vi "Arduino_Timed_Release.vi"(2 "Time to hold source ON (microseconds)":u32=1000000 format="%.0g", 3 "Time to hold source OFF (microseconds)":u32=1000000 format="%.0g", 4 "Number of cycles":u16=1) -> (0 "error out":errorcluster, 1 "Completed cycles":u16=5)   [LabVIEW 2022 SP3]
uses:
  ADAM Serial/Instrument drivers/Arduino/ctls_and_globals/Arduino Config & resource typedef.ctl
  ADAM Client/Sub VIs/ADAM Controls/Update_scan_value.ctl
  <vilib>/Utility/error.llb/Trim Whitespace One-Sided.vi
  Globals/Preference_global.vi
  Globals/Gas_management_global.vi
  Arduino_common/Arduino_comms_Global.vi
panel:
  out "element":T1={"baud rate (bps)"=276000, "timeout (ms)"=12000, "data bits"=8, "parity"=enum."None", "stop bits (10: 1 bit)"=10, "flow control"=0, "termination char (hex)"=10, "Enable Termination Char"=FALSE, "byte count"=12, "Resource locked?"=FALSE, "VISA resource name"=""} {"termination char (hex)" format="%02x"; "stop bits (10: 1 bit)" items=["1.0"=10, "1.5"=15, "2.0"=20]; "flow control" items=["None", "XON/XOFF", "RTS/CTS", "XON/XOFF & RTS/CTS", "DTR/DSR", "XON/XOFF & DTR/DSR"]}
  in  "Device index":i32
  out "bytes sent":u32=12
  out "write buffer":string
  # "(enter 0 for continuous ON)*"
  # "(enter 0 for continuous OFF)*"
  # "Paul Nathan, 18/06/2013, 02/05/2014, 12/08/2014, 03/10/2014, 10/12/2014"
  # "*until next communication. Ensure n cycles is 1 for these special operations."
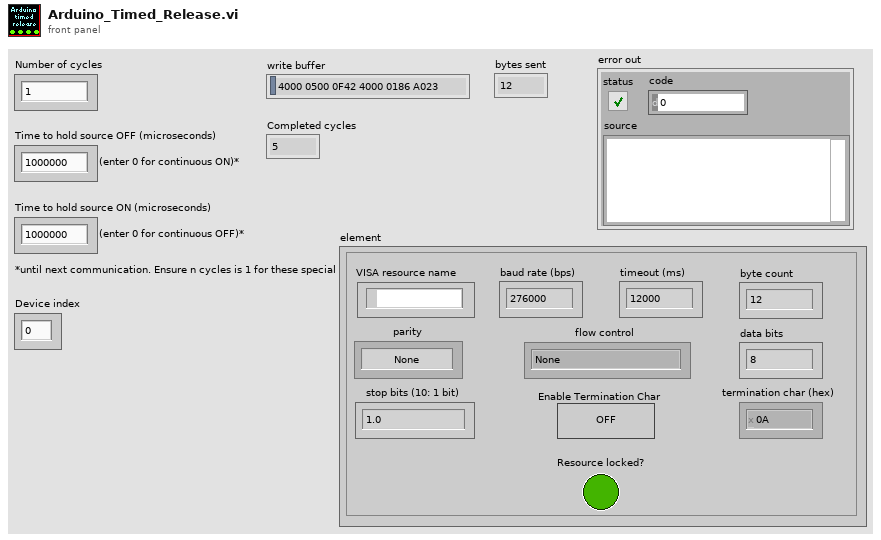
[diagram p1: front panel]
types:
  T1 = typedef "Arduino Config & resource typedef.ctl" = cluster{"baud rate (bps)":u32, "timeout (ms)":u32, "data bits":u16, "parity":enum16{"None", "Odd", "Even", "Mark", "Space"}, "stop bits (10: 1 bit)":u16, "flow control":u16, "termination char (hex)":u8, "Enable Termination Char":bool, "byte count":u32, "Resource locked?":bool, "VISA resource name":refnum<visa-resource-name>}
  T2 = cluster{"Rig Setup":string, "Device index":i32, "Number of cycles":u16, "Time to hold source OFF (microseconds)":u32, "Time to hold source ON (microseconds)":u32}
  T3 = typedef "Update_scan_value.ctl" = cluster{"Channel Name":string, "New Value":dbl, "!Auto_Off":bool}
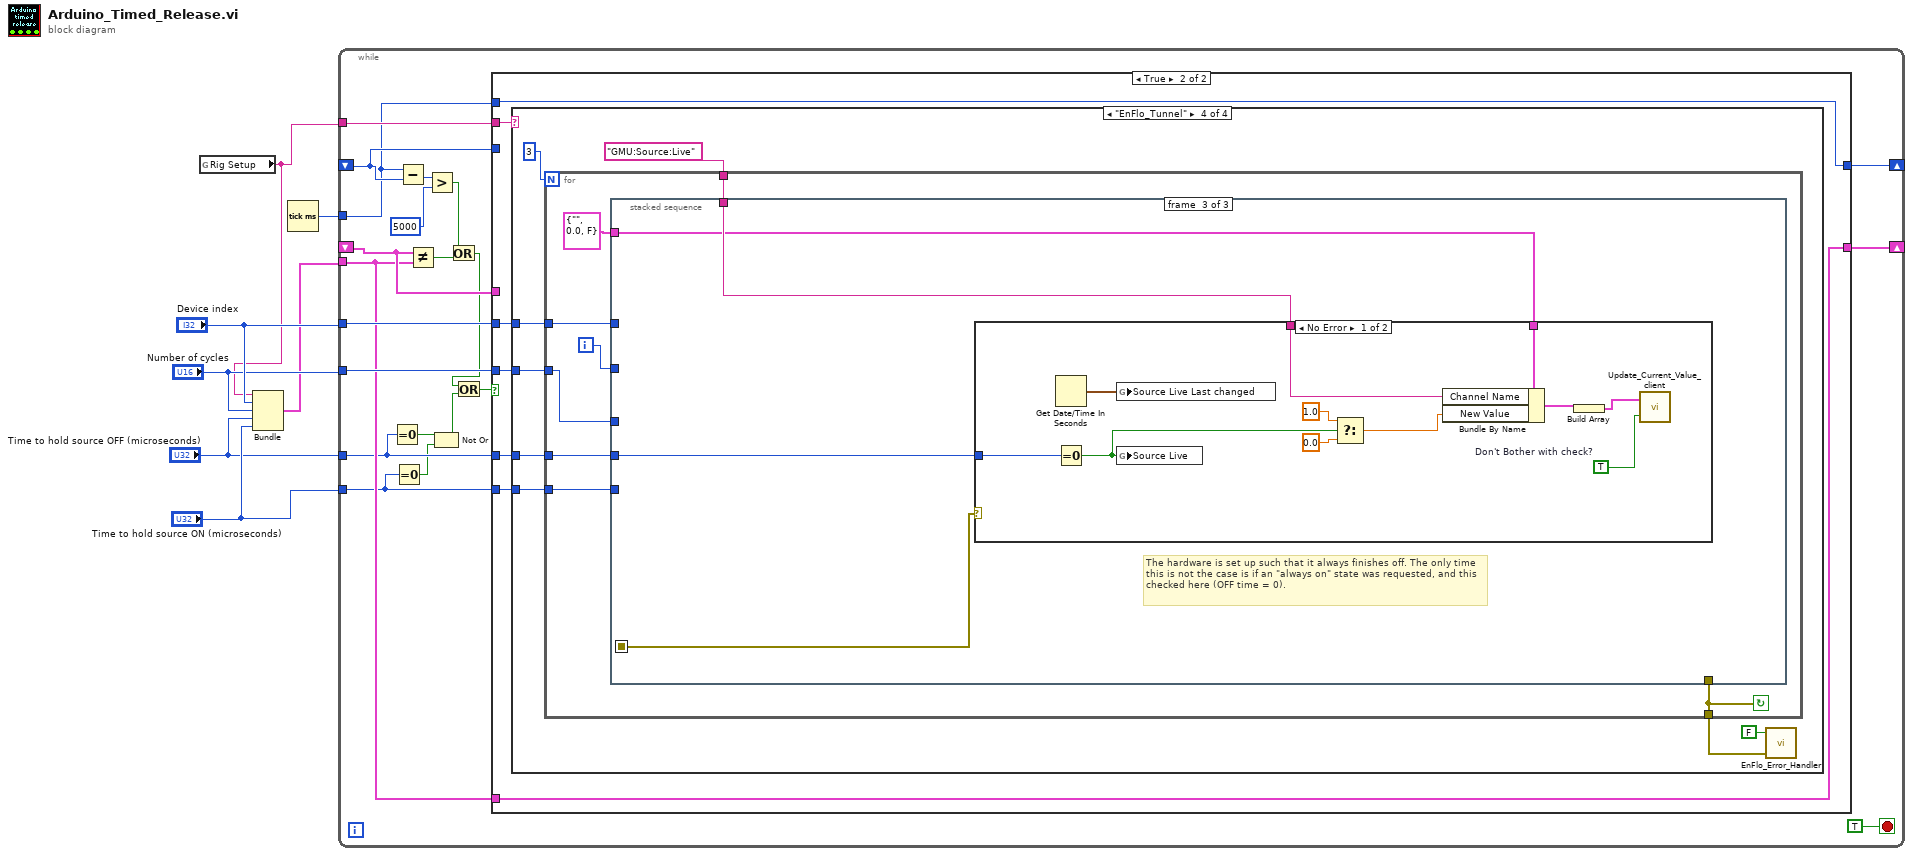
[diagram p0: block diagram]
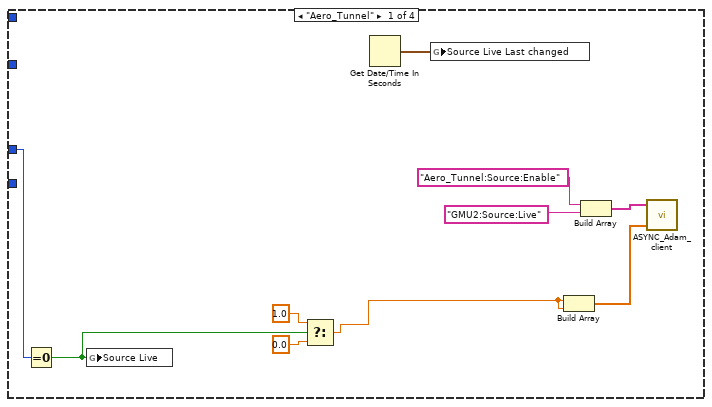
[diagram p3: hidden frame]
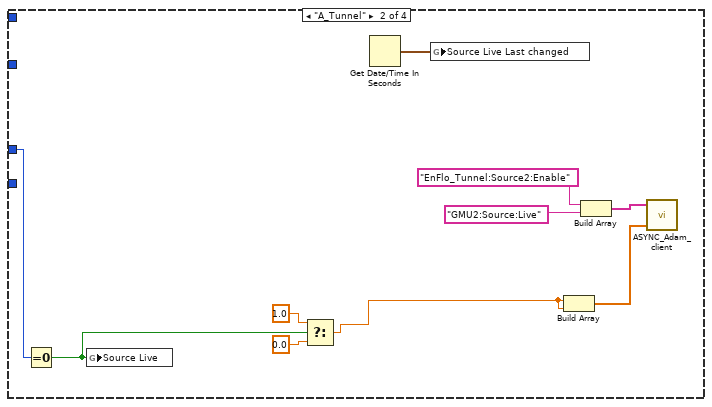
[diagram p4: hidden frame]
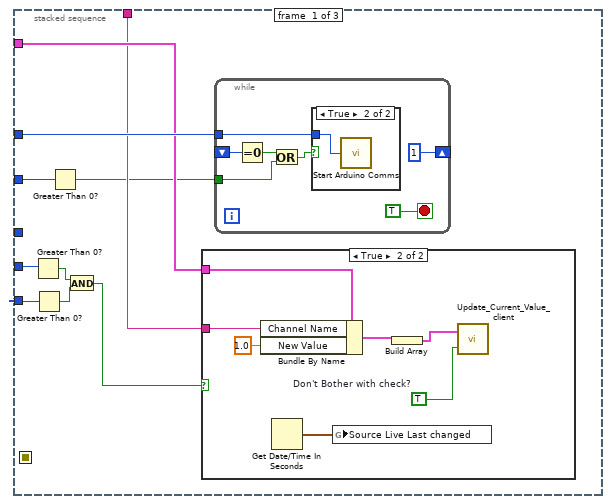
[diagram p6: hidden frame]
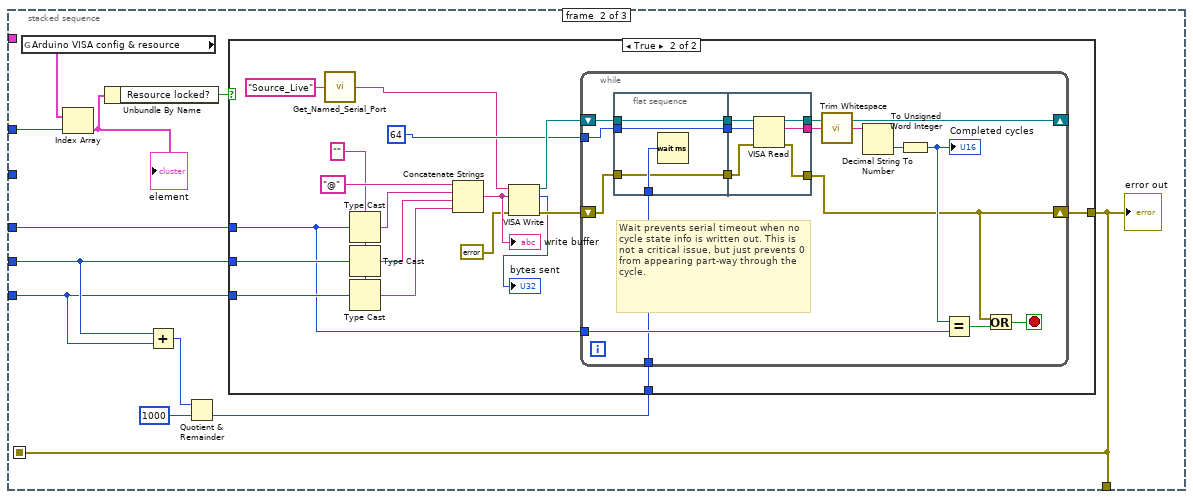
[diagram p9: hidden frame]
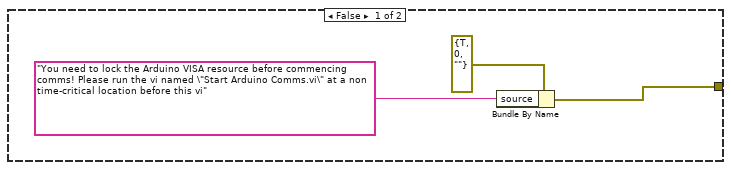
[diagram p10: hidden frame]
diagram:
  n1 = global read "Preference_global.vi" "Rig Setup"() -> (w4:string)
  n2 = Bundle("Rig Setup"=w4, "Device index"="Device index", "Number of cycles"="Number of cycles", "Time to hold source OFF (microseconds)"="Time to hold source OFF (microseconds)", "Time to hold source ON (microseconds)"="Time to hold source ON (microseconds)") -> (w5:T2)  [unwired: 1 in]
  n3 = Tick Count (ms)() -> (millisecond timer value=w3:u32)
  n4 = while {
    tunnel: "Device index" -> [w28]
    tunnel: "Number of cycles" -> [w27]
    tunnel: "Time to hold source ON (microseconds)" -> [w14]
    tunnel: "Time to hold source OFF (microseconds)" -> [w13]
    tunnel: w5 -> [w15]
    tunnel: w4 -> [w26]
    tunnel: w3 -> [w18]
    shift-right: [w17] -> _
    shift-left: _ -> [w16]
    shift-right: [w20] -> _
    shift-left: _ -> [w19]
    stop <- TRUE stop-if-true
    n5 = Equal To 0?(x=w13) -> (x = 0?=w12:bool)
    n6 = Equal To 0?(x=w14) -> (x = 0?=w11:bool)
    n7 = Subtract(x=w18, y=w19) -> (x-y=w25:u32)
    n8 = Not Equal?(x=w16, y=w15) -> (x != y?=w22:bool)
    n9 = Greater?(x=w25, y=u32 5000) -> (0:w23:bool)
    n10 = Not Or(1:w11, 2:w12) -> (0:w8:bool)
    n11 = Or(x=w23, y=w22) -> (x .or. y?=w10:bool)
    n12 = Or(x=w10, y=w8) -> (x .or. y?=w9:bool)
    n13 = case shown="True" w9 {
      tunnel: w26 -> [_ w37]
      tunnel: w28 -> [_ w36]
      tunnel: w27 -> [_ w35]
      tunnel: w14 -> [_ w34]
      tunnel: w13 -> [_ w33]
      tunnel: [w30 w32] -> w20
      tunnel: w19 -> [w30 _]
      tunnel: w18 -> [_ w32]
      tunnel: [w29 w31] -> w17
      tunnel: w16 -> [w29 _]
      tunnel: w15 -> [_ w31]
      frame False {
      }
      frame True {
        n14 = case shown="\"EnFlo_Tunnel\"" w37 {
          tunnel: w34 -> [_ _ _ w64]
          tunnel: w33 -> [w40 w50 _ w63]
          tunnel: w36 -> [_ _ _ w62]
          tunnel: w35 -> [_ _ _ w61]
          frame "Aero_Tunnel" {
            n15 = Equal To 0?(x=w40) -> (x = 0?=w43:bool)
            n16 = global write "Gas_management_global.vi" "Source Live"(w43) -> ()
            n17 = Select(t=1.0, s=w43, f=0.0) -> (s? t:f=w38:dbl)
            n18 = Get Date/Time In Seconds() -> (seconds since 1Jan1904=w44:timestamp)
            n19 = global write "Gas_management_global.vi" "Source Live Last changed"(w44) -> ()
            n20 = Build Array(w38, w38) -> (w47:dbl[])
            n21 = Build Array("Aero_Tunnel:Source:Enable", "GMU2:Source:Live") -> (w46:string[])
            n22 = call "ASYNC_Adam_client.vi"("Values"=w47, "Channel Names"=w46) -> ()  [unwired: 1 in, 2 out]
          }
          frame "A_Tunnel" {
            n23 = Equal To 0?(x=w50) -> (x = 0?=w53:bool)
            n24 = global write "Gas_management_global.vi" "Source Live"(w53) -> ()
            n25 = Select(t=1.0, s=w53, f=0.0) -> (s? t:f=w48:dbl)
            n26 = Get Date/Time In Seconds() -> (seconds since 1Jan1904=w54:timestamp)
            n27 = global write "Gas_management_global.vi" "Source Live Last changed"(w54) -> ()
            n28 = Build Array(w48, w48) -> (w57:dbl[])
            n29 = Build Array("EnFlo_Tunnel:Source2:Enable", "GMU2:Source:Live") -> (w56:string[])
            n30 = call "ASYNC_Adam_client.vi"("Values"=w57, "Channel Names"=w56) -> ()  [unwired: 1 in, 2 out]
          }
          frame Default {
          }
          frame "EnFlo_Tunnel" {
            n31 = for {
              N: 3 -> [_]
              tunnel: w64 -> [w69]
              tunnel: w63 -> [w70]
              tunnel: w62 -> [w72]
              tunnel: w61 -> [w71]
              tunnel: "GMU:Source:Live" -> [w68]
              tunnel: [w67] -> w58
              i -> [w66]
              stop <- w67 continue-if-true
              n32 = stacked-sequence {
                seq-local: [_ w99 _] -> [_ _ w157]
                tunnel: w72 -> [w83 w103 _]
                tunnel: w71 -> [_ w102 _]
                tunnel: w70 -> [w80 w101 w160]
                tunnel: w69 -> [w79 w100 _]
                tunnel: w68 -> [w81 _ w159]
                tunnel: T3 {"Channel Name"="", "New Value"=0.0, "!Auto_Off"=FALSE} ("Update Scan Value Cluster") -> [w82 _ w158]
                tunnel: [_ w99 _] -> w67
                tunnel: w66 -> [w75 _ _]
                frame #0 {
                  n33 = Greater Than 0?(x=w80) -> (x > 0?=w78:bool)
                  n34 = Greater Than 0?(x=w79) -> (x > 0?=w77:bool)
                  n35 = Greater Than 0?(x=w75) -> (x > 0?=w74:bool)
                  n36 = And(x=w78, y=w77) -> (x .and. y?=w76:bool)
                  n37 = case shown="True" w76 {
                    tunnel: w82 -> [_ w87]
                    tunnel: w81 -> [_ w86]
                    frame False {
                    }
                    frame True {
                      w88 = TRUE  # Don't Bother with check?
                      n38 = Bundle By Name(cluster=w87, "Channel Name"=w86, "New Value"=1.0) -> (w90:T3)
                      n39 = Get Date/Time In Seconds() -> (seconds since 1Jan1904=w84:timestamp)
                      n40 = global write "Gas_management_global.vi" "Source Live Last changed"(w84) -> ()
                      n41 = Build Array(w90) -> (w89:T3[])
                      n42 = call "Update_Current_Value_client.vi"("Don't Bother with check?"=w88, "Update array in"=w89) -> ()
                    }
                  }
                  n43 = while {
                    shift-right: [1] -> _
                    shift-left: _ -> [w97]
                    tunnel: w83 -> [w94]
                    tunnel: w74 -> [w91]
                    stop <- TRUE stop-if-true
                    n44 = Equal To 0?(x=w97) -> (x = 0?=w93:bool)
                    n45 = Or(x=w93, y=w91) -> (x .or. y?=w92:bool)
                    n46 = case shown="True" w92 {
                      tunnel: w94 -> [_ w98]
                      frame False {
                      }
                      frame True {
                        n47 = call "Start Arduino Comms.vi"("Resource index"=w98) -> ()  [unwired: 1 out]
                      }
                    }
                  }
                }
                frame #1 {
                  n48 = global read "Arduino_comms_Global.vi" "Arduino VISA config & resource"() -> (w105:T1[])
                  n49 = Index Array(array=w105, index=w103) -> (element=w104:T1)
                  "element" <- w104
                  n50 = Unbundle By Name(w104) -> ("Resource locked?"=w109:bool)
                  n51 = Add(x=w101, y=w100) -> (x+y=w108:u32)
                  n52 = Quotient & Remainder(x=w108, y=u32 1000) -> (floor(x/y)=w106:u32)  [unwired: 1 out]
                  n53 = case shown="True" w109 {
                    tunnel: w102 -> [_ w119]
                    tunnel: w101 -> [_ w127]
                    tunnel: w100 -> [_ w126]
                    tunnel: [w110 w121] -> w99
                    tunnel: w106 -> [_ w116]
                    frame False {
                      n54 = Bundle By Name(cluster=errorcluster {"status"=TRUE, "code"=0, "source"=""} ("error out"), "source"="You need to lock the Arduino VISA resource before commencing comms! Please run the vi named \"Start Arduino Comms.vi\" at a non time-critical location before this vi") -> (w110:errorcluster)
                    }
                    frame True {
                      w128 = ""
                      n55 = call "Get_Named_Serial_Port.vi"("Serial Port Alias"="Source_Live") -> ("Serial Port Name"=w113:string)
                      n56 = Type Cast(type=w128, x=w119) -> (*(type *) &x=w125:string)
                      n57 = Type Cast(type=w128, x=w127) -> (*(type *) &x=w124:string)
                      n58 = Type Cast(type=w128, x=w126) -> (*(type *) &x=w123:string)
                      n59 = Concatenate Strings("@", w125, w124, w123) -> (w129:string)
                      "write buffer" <- w129
                      n60 = VISA Write(VISA resource name=w113, write buffer=w129, error in (no error)=errorcluster {"status"=FALSE, "code"=0, "source"=""}) -> (VISA resource name out=w118:refnum<visa-resource-name>, return count=→"bytes sent":u32, error out=w122:errorcluster)
                      n61 = while {
                        tunnel: u32 64 ("byte count") -> [w145]
                        shift-right: [w133] -> w121
                        shift-left: w122 -> [w135]
                        shift-right: [w144] -> _
                        shift-left: w118 -> [w146]
                        tunnel: w119 -> [w142]
                        tunnel: w116 -> [w136]
                        stop <- w131 stop-if-true
                        # "Wait prevents serial timeout when no cycle state info is written out. This is not a critical issue, but just prevents 0 from appearing part-way through the cycle."
                        n62 = flat-sequence {
                          tunnel: w145 -> [w149]
                          tunnel: w146 -> [w150]
                          tunnel: [w150] -> w138
                          tunnel: [w149] -> w137
                          tunnel: w136 -> [w148]
                          tunnel: w135 -> [w147]
                          tunnel: [w147] -> w134
                          tunnel: [w154] -> w144
                          tunnel: [w153] -> w140
                          tunnel: w138 -> [w156]
                          tunnel: w137 -> [w155]
                          tunnel: w134 -> [w152]
                          tunnel: [w151] -> w133
                          frame #0 {
                            n63 = Wait (ms)(milliseconds to wait=w148) -> ()  [unwired: 1 out]
                          }
                          frame #1 {
                            n64 = VISA Read(VISA resource name=w156, byte count=w155, error in (no error)=w152) -> (VISA resource name out=w154:refnum<visa-resource-name>, read buffer=w153:string, error out=w151:errorcluster)  [unwired: 1 out]
                          }
                        }
                        n65 = call <vilib>:"Trim Whitespace.vi"("string"=w140) -> ("trimmed string"=w139:string)  [unwired: 1 in]
                        n66 = Decimal String To Number(string=w139) -> (number=w143:i32)  [unwired: 2 in, 1 out]
                        n67 = To Unsigned Word Integer(number=w143) -> (unsigned 16bit integer=w141:u16)
                        "Completed cycles" <- w141
                        n68 = Equal?(x=w141, y=w142) -> (x = y?=w132:bool)
                        n69 = Or(x=w133, y=w132) -> (x .or. y?=w131:bool)
                      }
                    }
                  }
                  "error out" <- w99
                }
                frame #2 {
                  # "The hardware is set up such that it always finishes off. The only time this is not the case is if an \"always on\" state was requested, and this checked here (OFF time = 0)."
                  n70 = case shown="No Error" w157 {
                    tunnel: w160 -> [w170 _]
                    tunnel: w159 -> [w162 _]
                    tunnel: w158 -> [w161 _]
                    frame No Error {
                      w163 = TRUE  # Don't Bother with check?
                      n71 = Get Date/Time In Seconds() -> (seconds since 1Jan1904=w171:timestamp)
                      n72 = Equal To 0?(x=w170) -> (x = 0?=w169:bool)
                      n73 = global write "Gas_management_global.vi" "Source Live Last changed"(w171) -> ()
                      n74 = global write "Gas_management_global.vi" "Source Live"(w169) -> ()
                      n75 = Select(t=1.0, s=w169, f=0.0) -> (s? t:f=w166:dbl)
                      n76 = Bundle By Name(cluster=w161, "Channel Name"=w162, "New Value"=w166) -> (w165:T3)
                      n77 = Build Array(w165) -> (w164:T3[])
                      n78 = call "Update_Current_Value_client.vi"("Don't Bother with check?"=w163, "Update array in"=w164) -> ()
                    }
                    frame Error {
                    }
                  }
                }
              }
            }
            n79 = call "EnFlo_Error_Handler.vi"("error in (no error)"=w58, "Dialog Box (F)"=FALSE ("Dialog Box (T)")) -> ()  [unwired: 2 in, 2 out]
          }
        }
      }
    }
  }
